vi "LVClass_SlopesPostProcessList GetParameter_Pupil.vi"(0 "SlopesPostProcessorList in":refnum<class "SlopesPostProcessorList.lvclass">, 5 "Position":u32, 7 "Pupil.lvclass":refnum<class "Pupil.lvclass">, 11 "error in (no error)":errorcluster) -> (4 "SlopesPostProcessorList out":refnum<class "SlopesPostProcessorList.lvclass">, 8 "Pupil Out":refnum<class "Pupil.lvclass">, 10 "Comment":string, 15 "error out":errorcluster)   [LabVIEW 2020, in "SlopesPostProcessorList.lvclass"]
doc: "Get parameters of the Pupil processor.\n\n--------------------------------------------------------------------------------\n\n<B>SlopesPostProcessorListIn </B> : SlopesPostProcessorList object.\n<B>SlopesPostProcessorListOut </B> : SlopesPostProcessorList object.\n<B>position </B> : Position of the processor in the SlopesPostProcessorList.\n<B>Pupil </B> : pupil object.\n<B>ErrorIn </B> : Error\n<B>ErrorOut </B> : Error\n\n--------------------------------------------------------------------------------"
uses:
  SlopesPostProcessorList.lvclass
  Pupil.lvclass
  SlopesPostProcessorList.lvclass/SlopesPostProcessorList.ctl
  LVClass_Pupil Read Pupil.vi
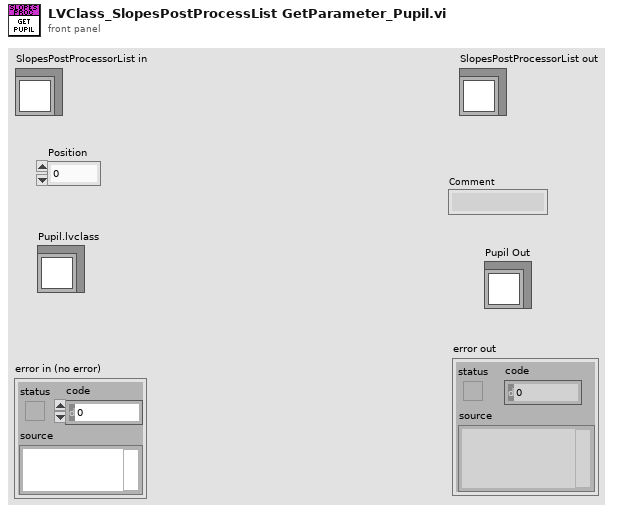
[diagram p1: front panel]
types:
  T1 = typedef "General dimensions definition.ctl" = cluster{"Size":T2, "Step":T3}
  T2 = typedef "Point2D.ctl" = cluster{"X":u32, "Y":u32}
  T3 = typedef "Point2Df.ctl" = cluster{"X":sgl, "Y":sgl}
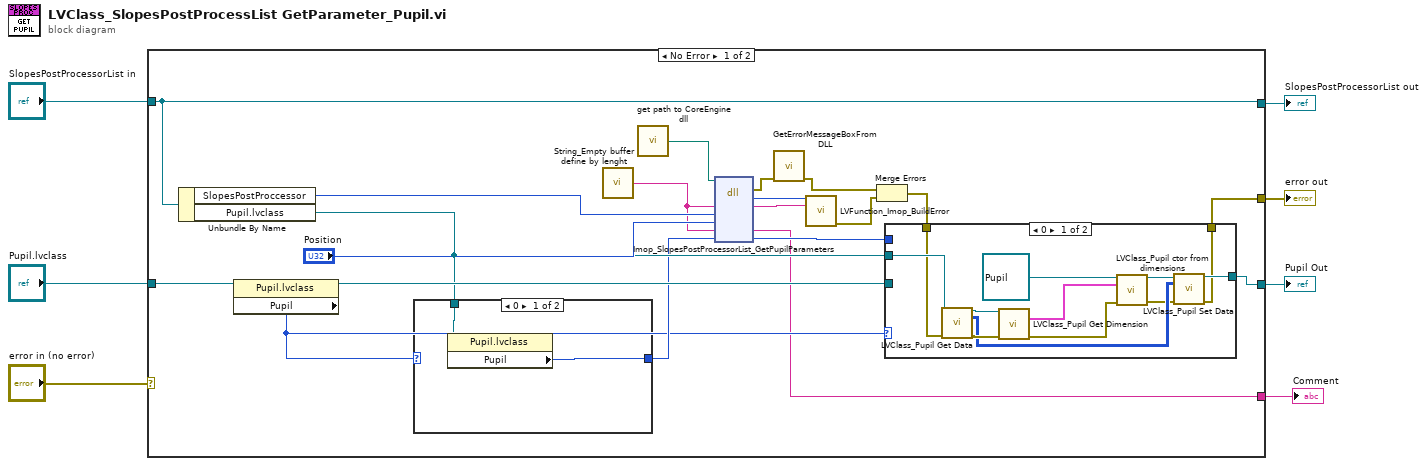
[diagram p0: block diagram]
diagram:
  n1 = case shown="No Error" "error in (no error)" {
    selector: "error in (no error)" -> [_ w46]
    tunnel: "SlopesPostProcessorList in" -> [w23 w47]
    tunnel: [w23 w47] -> w5
    tunnel: [w17 w46] -> w4
    tunnel: "Pupil.lvclass" -> [w20 w45]
    tunnel: [w16 w45] -> w2
    tunnel: [w9 _] -> w1
    frame No Error {
      n2 = Unbundle By Name(w23) -> ("SlopesPostProccessor"=w22:i32, "Pupil.lvclass"=w13:refnum<class "Pupil.lvclass">)
      n3 = property class="Pupil.lvclass"(reference=w20) -> (reference out=w15:refnum<class "Pupil.lvclass">, "Pupil"=w10:i32)  [unwired: 1 in, 1 out]
      n4 = case shown="0" w10 {
        selector: w10 -> [_ w44]
        tunnel: w13 -> [w43 _]
        tunnel: [w42 w44] -> w11
        frame 0 {
          n5 = property class="Pupil.lvclass"(reference=w43) -> ("Pupil"=w42:i32)  [unwired: 1 in, 2 out]
        }
        frame 1, Default {
        }
      }
      n6 = call "String_Empty buffer define by lenght.vi"() -> ("Empty buffer"=w8:string)  [unwired: 1 in]
      n7 = call "get path to CoreEngine dll.vi"() -> ("path to c_interface_vc100.dll"=w25:path)  [unwired: 12 in, 3 out]
      n8 = dll-call lib="D:/soft/HASO_v3/SVN_trunk/ImOpCoreEngine4_LV2011/DLLs/c_interface_vc100.dll" fn="Imop_SlopesPostProcessorList_GetPupilParameters"(path in=w25, "message"=w8, "objet"=w22, "Position"="Position", "Pupil file path"=w8, "pupil"=w11) -> (error out=w24:errorcluster, "return type"=w26:i32, "message"=w27:string, "Pupil file path"=w9:string, "pupil"=w14:i32)  [unwired: 4 in, 1 out]
      n9 = call "GetErrorMessageBoxFromDLL.vi"("error IN"=w24) -> ("error OUT"=w19:errorcluster)  [unwired: 10 in]
      n10 = call "LVFunction_Imop_BuildError.vi"("code"=w26, "String to Prepend to source (\"\")"=w27) -> ("error out"=w18:errorcluster)  [unwired: 13 in]
      n11 = Merge Errors(w19, w18) -> (w12:errorcluster)
      n12 = case shown="0" w10 {
        tunnel: w13 -> [w34 _]
        tunnel: [w36 w41] -> w16
        tunnel: w15 -> [_ w41]
        tunnel: w12 -> [w32 w40]
        tunnel: [w29 w40] -> w17
        tunnel: w14 -> [_ _]
        frame 0 {
          n13 = call "LVClass_Pupil Get Data.vi"("Pupil in"=w34, "error in (no error)"=w32) -> ("Pupil out"=w33:refnum<class "Pupil.lvclass">, "Data"=w30:i32[][], "error out"=w31:errorcluster)  [unwired: 11 in]
          n14 = call "LVClass_Pupil Get Dimension.vi"("Pupil in"=w33, "error in (no error)"=w31) -> ("Dimension"=w39:T1, "error out"=w35:errorcluster)  [unwired: 11 in, 1 out]
          n15 = call "LVClass_Pupil ctor from dimensions.vi"("Pupil in"=refnum<class "Pupil.lvclass"> refnum, "Dimensions_um"=w39, "error in (no error)"=w35) -> ("Pupil out"=w37:refnum<class "Pupil.lvclass">, "error out"=w28:errorcluster)  [unwired: 11 in]
          n16 = call "LVClass_Pupil Set Data.vi"("Pupil in"=w37, "Data"=w30, "error in (no error)"=w28) -> ("Pupil out"=w36:refnum<class "Pupil.lvclass">, "error out"=w29:errorcluster)  [unwired: 11 in]
        }
        frame 1, Default {
        }
      }
    }
    frame Error {
    }
  }
  "error out" <- w4
  "SlopesPostProcessorList out" <- w5
  "Pupil Out" <- w2
  "Comment" <- w1
